vi "Convert Temperature.vi"(3 "Temperature (deg C)":dbl, 5 "error in (no error)":errorcluster) -> (16 "Temperature (deg F)":dbl, 19 "error out":errorcluster)   [LabVIEW 2017, in "Temp.lvclass"]
uses:
  Temp.lvclass
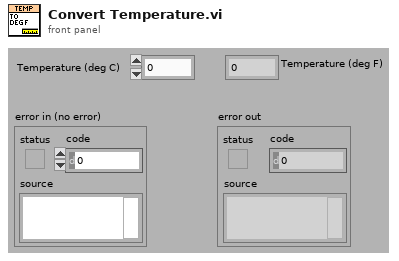
[diagram p1: front panel]
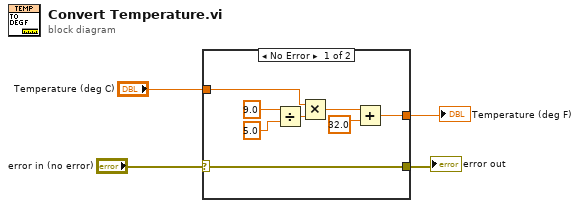
[diagram p0: block diagram]
diagram:
  n1 = case shown="No Error" "error in (no error)" {
    selector: "error in (no error)" -> [w5 w13]
    tunnel: [w5 w13] -> w3
    tunnel: "Temperature (deg C)" -> [w7 _]
    tunnel: [w6 _] -> w1
    frame No Error {
      n2 = Divide(x=9.0, y=5.0) -> (x/y=w10:dbl)
      n3 = Multiply(x=w7, y=w10) -> (x*y=w9:dbl)
      n4 = Add(x=w9, y=32.0) -> (x+y=w6:dbl)
    }
    frame Error {
    }
  }
  "error out" <- w3
  "Temperature (deg F)" <- w1
